vi "Create APU Register Bus.vi"(11 "shared settings.<user name>":T1 {"start" format="%#.15g"}) -> (3 "register bus":T2={"Speed"="Speed", "Crank Angle"="Crank Angle", "Cycle Angle"="Cycle Angle", "Crank Count"="Crank Count", "Cycle Count"="Cycle Count", "1.25 MHz Counter"="1.25 MHz Counter", "Crank Rollover"="Crank Rollover", "Cycle Rollover"="Cycle Rollover", "shared settings"={"start"=0.0, "stuck limit"=0.0}} {"shared settings"."start" format="%#.15g"})   [LabVIEW 2015, in "Engine Simulation Toolkit.lvlib" / "APU.lvlib"]
doc: "Creates the <b>register bus</b> for all components linked to this APU. Place this VI on the root diagram of your FPGA VI and wire the <b>register bus</b> to all components you want sharing speed and position data."
uses:
  APU.lvlib
  Register Bus.ctl
  Shared Settings.ctl
  <vilib>/rvi/DataTransferAndStorage/Container/Common/niFpgaContainerGetUniqueNameForEmu.vi
  <vilib>/rvi/DataTransferAndStorage/Container/Common/niFpgaContainerSetEmuInfo.vi
  <vilib>/rvi/eio/common/nirviEmuReportErrorAndStop.vi
  <vilib>/rvi/LocalResourceManager/LocalResourceManager.xnode
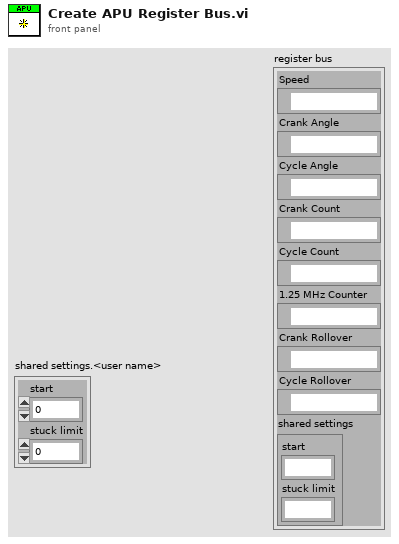
[diagram p1: front panel]
types:
  T1 = typedef "Engine Simulation Toolkit.lvlib/APU.lvlib/Shared Settings.ctl" = cluster{"start":fxp<+,17,17>, "stuck limit":fxp<+,18,18>}
  T2 = typedef "Engine Simulation Toolkit.lvlib/APU.lvlib/Register Bus.ctl" = cluster{"Speed":refnum<k21>, "Crank Angle":refnum<k21>, "Cycle Angle":refnum<k21>, "Crank Count":refnum<k21>, "Cycle Count":refnum<k21>, "1.25 MHz Counter":refnum<k21>, "Crank Rollover":refnum<k21>, "Cycle Rollover":refnum<k21>, "shared settings":T1}
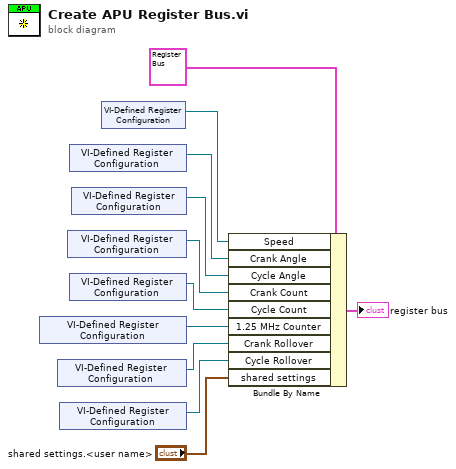
[diagram p0: block diagram]
diagram:
  n1 = xnode ("VI-Defined Register Configuration")() -> ("Register Out"=w4:refnum<k21>)
  n2 = xnode ("VI-Defined Register Configuration")() -> ("Register Out"=w2:refnum<k21>)
  n3 = xnode ("VI-Defined Register Configuration")() -> ("Register Out"=w1:refnum<k21>)
  n4 = xnode ("VI-Defined Register Configuration")() -> ("Register Out"=w6:refnum<k21>)
  n5 = xnode ("VI-Defined Register Configuration")() -> ("Register Out"=w8:refnum<k21>)
  n6 = xnode ("VI-Defined Register Configuration")() -> ("Register Out"=w5:refnum<k21>)
  n7 = xnode ("VI-Defined Register Configuration")() -> ("Register Out"=w7:refnum<k21>)
  n8 = xnode ("VI-Defined Register Configuration")() -> ("Register Out"=w9:refnum<k21>)
  n9 = Bundle By Name(cluster=T2 {"Speed"="", "Crank Angle"="", "Cycle Angle"="", "Crank Count"="", "Cycle Count"="", "1.25 MHz Counter"="", "Crank Rollover"="", "Cycle Rollover"="", "shared settings"={"start"=0.0, "stuck limit"=0.0}} ("register bus local output v1.0.0"), "Speed"=w9, "Crank Angle"=w8, "Cycle Angle"=w7, "Crank Count"=w6, "Cycle Count"=w5, "1.25 MHz Counter"=w4, "Crank Rollover"=w2, "Cycle Rollover"=w1, "shared settings"="shared settings.<user name>") -> (→"register bus":T2)
